vi "validate key value pair.vi"(8 "error in":errorcluster, 9 "value":string, 10 "key":string, 11 "CentralErrorHandlerDev configuration in":refnum<class "CentralErrorHandler configuration.lvclass">) -> (0 "error out":errorcluster, 3 "CentralErrorHandlerDev configuration out":refnum<class "CentralErrorHandler configuration.lvclass">)   [LabVIEW 2017, in "CentralErrorHandler configuration.lvclass"]
uses:
  CentralErrorHandler configuration.lvclass
  <vilib>/NI/DCAF/Tag Editor Core/control module/configuration/control module configuration.lvclass
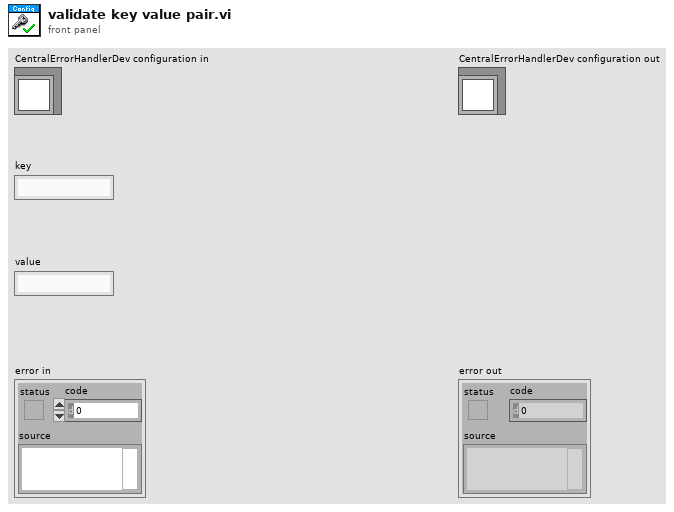
[diagram p1: front panel]
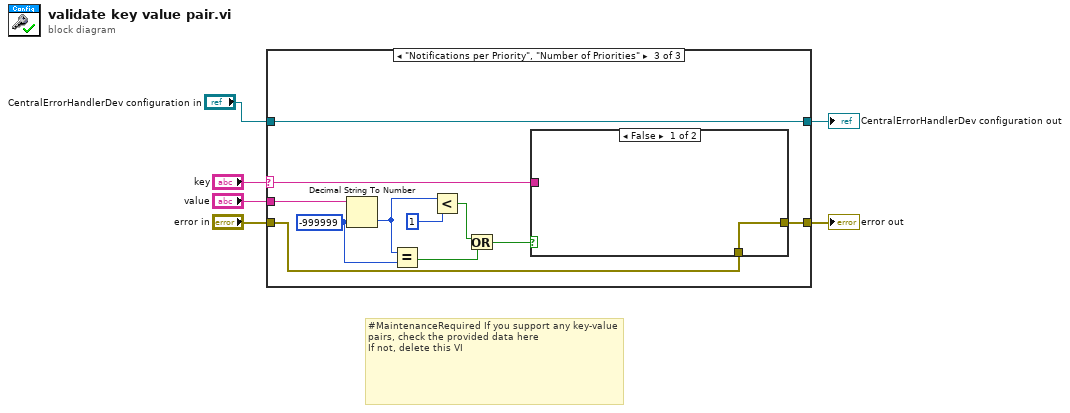
[diagram p0: block diagram]
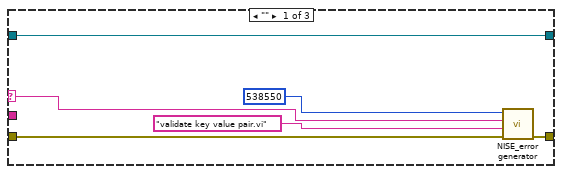
[diagram p2: hidden frame]
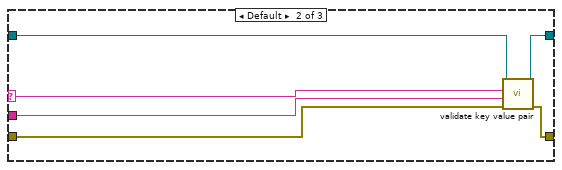
[diagram p3: hidden frame]
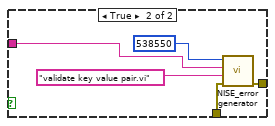
[diagram p4: hidden frame]
diagram:
  # "#MaintenanceRequired If you support any key-value pairs, check the provided data here\nIf not, delete this VI"
  n1 = case shown="\"Notifications per Priority\", \"Number of Priorities\"" "key" {
    selector: "key" -> [w9 w13 w22]
    tunnel: [w7 w18 w20] -> w6
    tunnel: [w12 w17 w23] -> w5
    tunnel: "error in" -> [w8 w16 w21]
    tunnel: "value" -> [_ w15 w29]
    tunnel: "CentralErrorHandlerDev configuration in" -> [w12 w14 w23]
    frame "" {
      n2 = call <vilib>:"NISE_error generator.vi"("error in"=w8, "source"="validate key value pair.vi", "append error message"=w9, "error code (0)"=538550) -> ("error out"=w7:errorcluster)  [unwired: 5 in]
    }
    frame Default {
      n3 = call-parent "validate key value pair.vi"("error in"=w16, "value"=w15, "key"=w13, "fixed channel configuration in"=w14) -> ("error out"=w18:errorcluster, "fixed channel configuration out"=w17:refnum<class "CentralErrorHandler configuration.lvclass">)  [unwired: 6 in]
    }
    frame "Notifications per Priority", "Number of Priorities" {
      w28 = -999999 ("default (0 I32)")
      n4 = Decimal String To Number(string=w29, default (0L)=w28) -> (number=w27:i32)  [unwired: 1 in, 1 out]
      n5 = Equal?(x=w27, y=w28) -> (x = y?=w24:bool)
      n6 = Less?(x=w27, y=1) -> (x < y?=w25:bool)
      n7 = Or(x=w25, y=w24) -> (x .or. y?=w19:bool)
      n8 = case shown="False" w19 {
        tunnel: w22 -> [_ w33]
        tunnel: w21 -> [w30 w32]
        tunnel: [w30 w31] -> w20
        frame False {
        }
        frame True {
          n9 = call <vilib>:"NISE_error generator.vi"("error in"=w32, "source"="validate key value pair.vi", "append error message"=w33, "error code (0)"=538550) -> ("error out"=w31:errorcluster)  [unwired: 5 in]
        }
      }
    }
  }
  "error out" <- w6
  "CentralErrorHandlerDev configuration out" <- w5
